vi "simple_publisher_event.vi"() -> ()   [LabVIEW 2014]
panel:
  in  "停止":bool
  in  "发送":bool
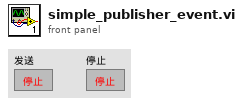
[diagram p1: front panel]
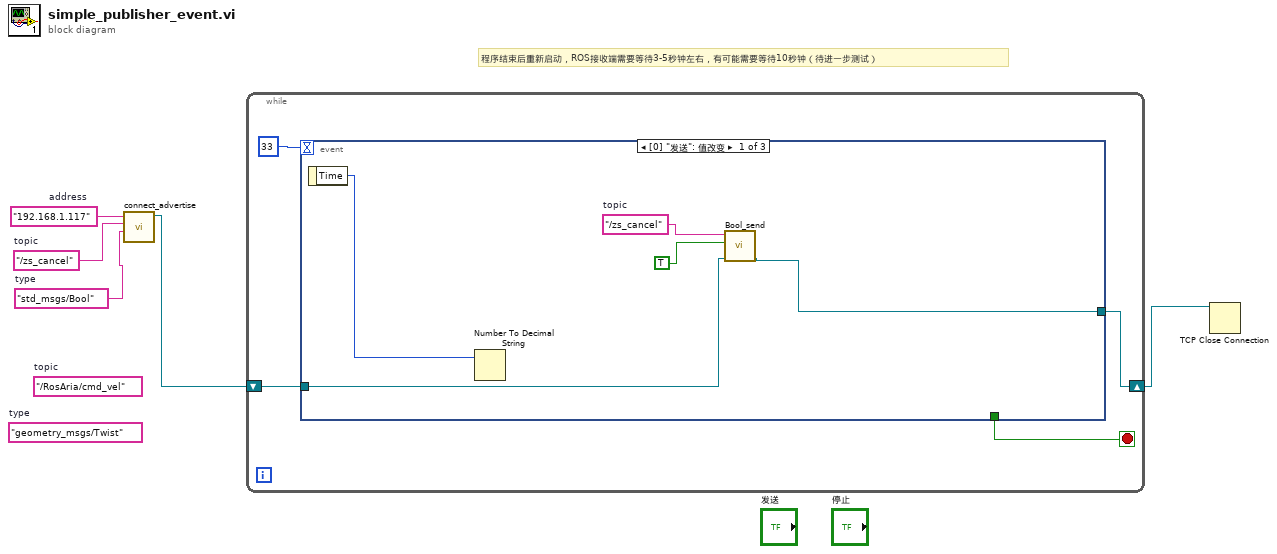
[diagram p0: block diagram]
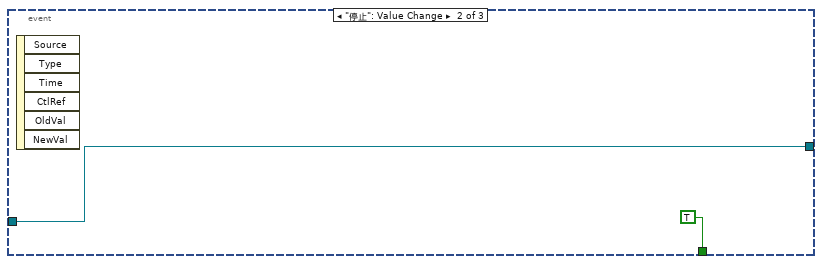
[diagram p2: hidden frame]
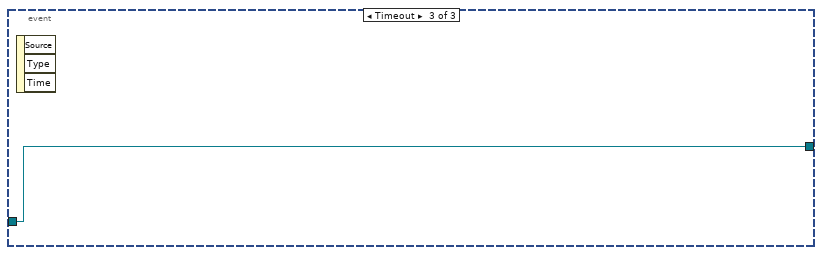
[diagram p3: hidden frame]
diagram:
  w4 = "192.168.1.117"  # address
  w2 = "std_msgs/Bool"  # type
  w3 = "/zs_cancel"  # topic
  (unwired) "geometry_msgs/Twist"  # type
  (unwired) "/RosAria/cmd_vel"  # topic
  # "程序结束后重新启动，ROS接收端需要等待3-5秒钟左右，有可能需要等待10秒钟（待进一步测试）"
  n1 = call "connect_advertise.vi"("type"=w2, "topic"=w3, "address"=w4) -> ("连接ID输出"=w1:refnum<k5>)  [unwired: 7 in, 1 out]
  n2 = while {
    shift-right: [w7] -> w5
    shift-left: w1 -> [w6]
    stop <- w8 stop-if-true
    n3 = event shown="[0] \"发送\": 值改变" {
      selector: _ -> [_ _ _]
      dyn-events: _ -> [_ _ _]
      timeout: 33 -> [_ _ _]
      tunnel: [_ TRUE _] -> w8
      tunnel: [w10 w15 w17] -> w7
      tunnel: w6 -> [w12 w15 w17]
      event "发送": Value Change {
        w13 = "/zs_cancel"  # topic
        n4 = event-data() -> ("Time"=w14:u32)  [unwired: 1 in]
        n5 = Number To Decimal String(number=w14) -> ()  [unwired: 1 in, 1 out]
        n6 = call "Bool_send.vi"("连接ID"=w12, "msg.data"=TRUE, "topic"=w13) -> ("连接ID输出"=w10:refnum<k5>)  [unwired: 8 in]
      }
      event "停止": Value Change {
        n7 = event-data() -> ()  [unwired: 1 in, 6 out]
      }
      event Timeout {
        n8 = event-data() -> ()  [unwired: 1 in, 3 out]
      }
    }
  }
  n9 = TCP Close Connection(connection ID=w5) -> ()  [unwired: 2 in, 2 out]
